vi "Traffic Control System.vi"() -> ()   [LabVIEW 2013]
panel:
  out "Red":bool
  out "Yellow":bool
  out "Green":bool
  in  "Dial 4":u16(knob) scale=0.0..9.0
  in  "Dial 3":u16(knob) scale=0.0..9.0
  in  "Dial 2":u16(knob) scale=0.0..9.0
  in  "Dial":u16(knob) scale=0.0..9.0
  in  "Yellow Timer (s)":u32
  in  "Red-Green Timer (s)":u32
  in  "Stop Button":bool
  out "Barricade Closed?":bool
  out "Barricade Open?":bool
  in  "Light State":enum16{"Red", "Green", "Yellow"}(ring)
  # "Timer Administration"
  # "Current Light State"
  # "Set the dials to correct position to enable timer modification controls"
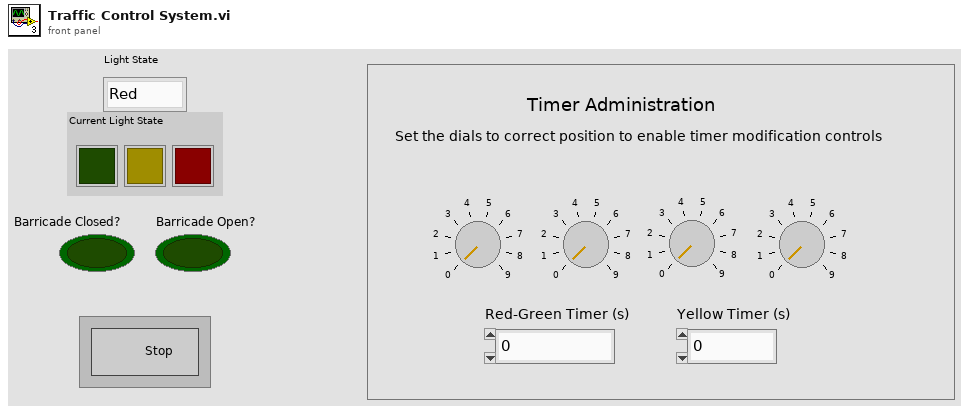
[diagram p1: front panel]
types:
  T1 = enum8{"Enabled", "Disabled", "Disabled and Grayed Out"}
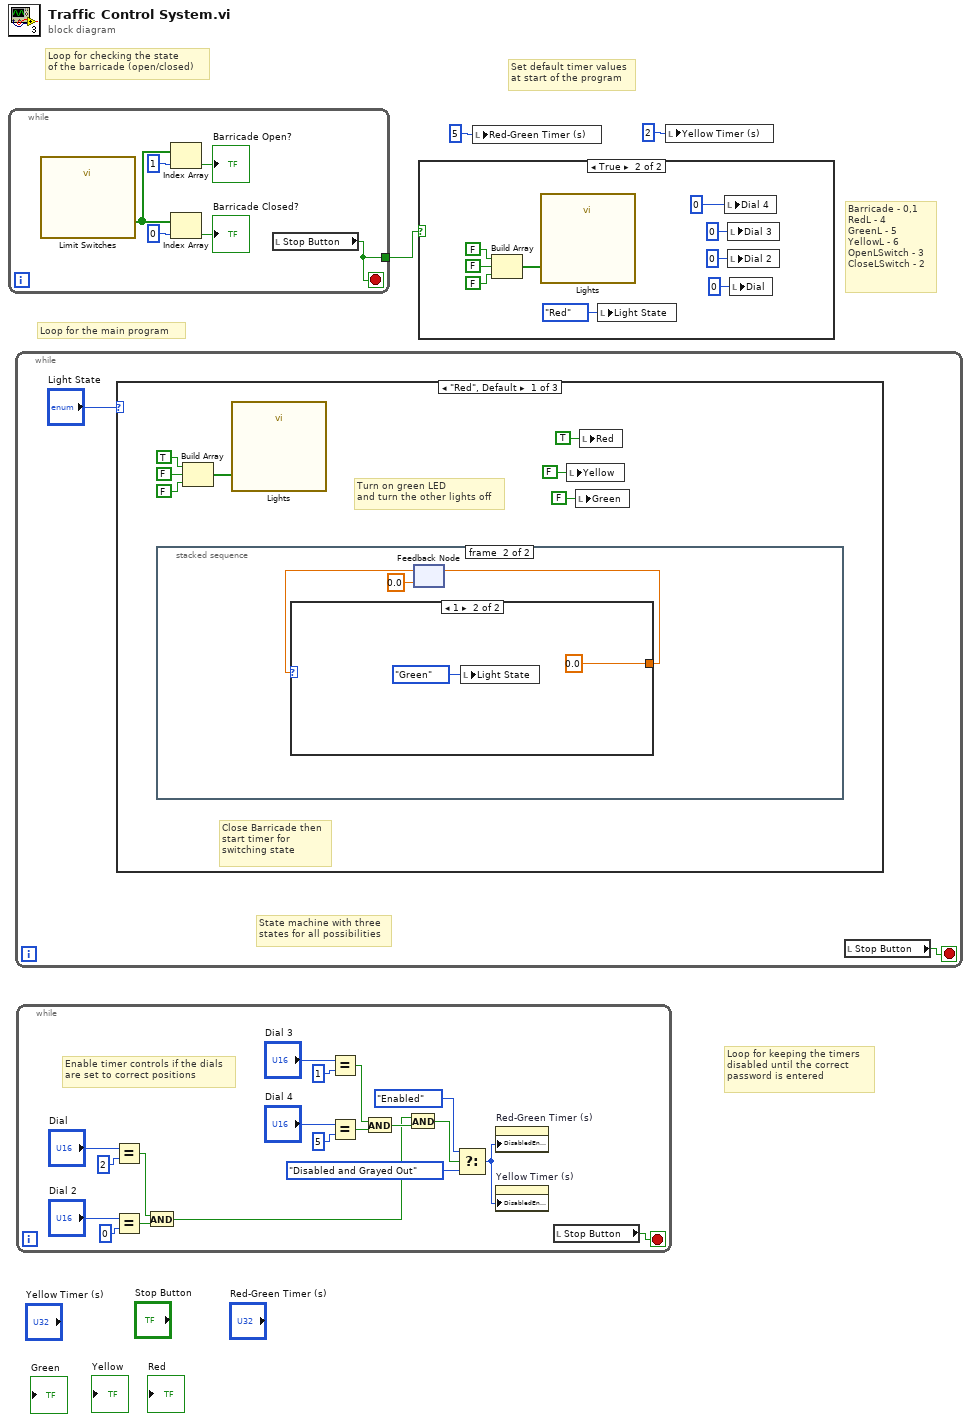
[diagram p0: block diagram]
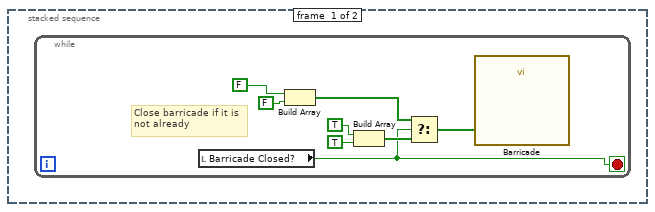
[diagram p3: hidden frame]
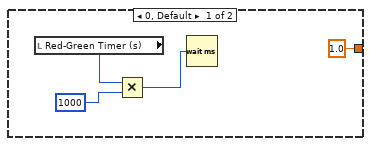
[diagram p4: hidden frame]
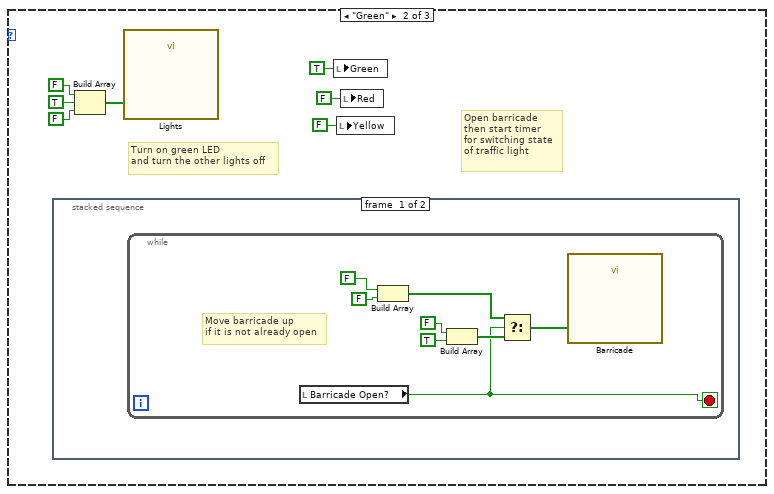
[diagram p5: hidden frame]
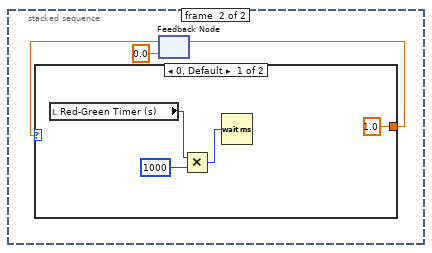
[diagram p6: hidden frame]
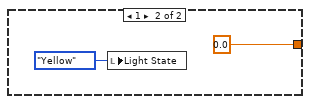
[diagram p7: hidden frame]
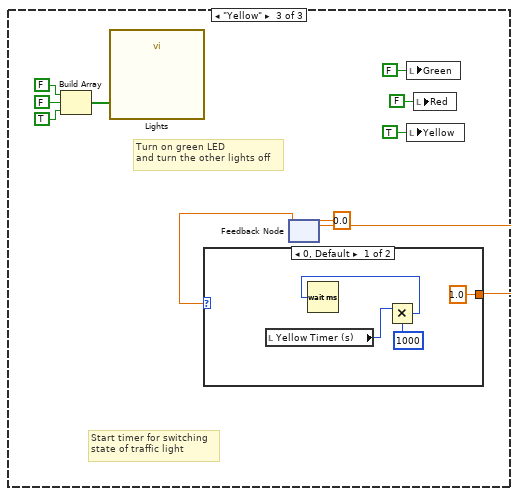
[diagram p8: hidden frame]
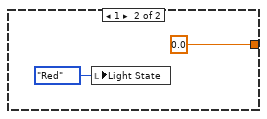
[diagram p9: hidden frame]
diagram:
  # "Loop for checking the state\nof the barricade (open/closed)"
  # "Loop for keeping the timers\ndisabled until the correct\npassword is entered"
  # "Set default timer values\nat start of the program"
  # "Loop for the main program"
  # "Barricade - 0,1\nRedL - 4\nGreenL - 5\nYellowL - 6\nOpenLSwitch - 3\nCloseLSwitch - 2"
  n1 = while {
    tunnel: [w4] -> w1
    stop <- w4 stop-if-true
    n2 = call "Limit Switches"() -> ("data"=w9:bool[])  [unwired: 17 in, 2 out]
    n3 = Index Array(array=w9, index=1) -> (element=→"Barricade Open?":bool)
    n4 = Index Array(array=w9, index=0) -> (element=→"Barricade Closed?":bool)
    n5 = local read "Stop Button"() -> (w4:bool)
  }
  n6 = while {
    stop <- w10 stop-if-true
    # "State machine with three\nstates for all possibilities"
    n7 = case shown="\"Red\", Default" "Light State" {
      frame "Red", Default {
        # "Turn on green LED\nand turn the other lights off"
        # "Close Barricade then\nstart timer for\nswitching state"
        n8 = stacked-sequence {
          frame #0 {
            n9 = while {
              stop <- w19 stop-if-true
              # "Close barricade if it is\nnot already"
              n10 = local read "Barricade Closed?"() -> (w19:bool)
              n11 = Build Array(FALSE, FALSE) -> (w21:bool[])
              n12 = Build Array(TRUE, TRUE) -> (w24:bool[])
              n13 = Select(t=w21, s=w19, f=w24) -> (s? t:f=w20:bool[])
              n14 = call "Barricade"("data"=w20) -> ()  [unwired: 17 in, 2 out]
            }
          }
          frame #1 {
            n15 = feedback #1(0.0) -> (w28:dbl)
            n16 = case shown="1" w28 {
              tunnel: [1.0 0.0] -> w29
              frame 0, Default {
                n17 = local read "Red-Green Timer (s)"() -> (w32:u32)
                n18 = Multiply(x=w32, y=u32 1000) -> (x*y=w30:u32)
                n19 = Wait (ms)(milliseconds to wait=w30) -> ()  [unwired: 1 out]
              }
              frame 1 {
                n20 = local write "Light State"(enum16{"Red", "Green", "Yellow"}."Green" ("Light State")) -> ()
              }
            }
            n21 = feedback-in #1(w29) -> ()
          }
        }
        n22 = Build Array(TRUE, FALSE, FALSE) -> (w15:bool[])
        n23 = call "Lights"("data"=w15) -> ()  [unwired: 17 in, 2 out]
        n24 = local write "Yellow"(FALSE ("Yellow")) -> ()
        n25 = local write "Green"(FALSE ("Green")) -> ()
        n26 = local write "Red"(TRUE ("Red")) -> ()
      }
      frame "Green" {
        # "Open barricade \nthen start timer\nfor switching state\nof traffic light"
        # "Turn on green LED\nand turn the other lights off"
        n27 = stacked-sequence {
          frame #0 {
            n28 = while {
              stop <- w43 stop-if-true
              # "Move barricade up\nif it is not already open"
              n29 = local read "Barricade Open?"() -> (w43:bool)
              n30 = Build Array(FALSE, FALSE) -> (w45:bool[])
              n31 = Build Array(FALSE, TRUE) -> (w48:bool[])
              n32 = Select(t=w45, s=w43, f=w48) -> (s? t:f=w44:bool[])
              n33 = call "Barricade"("data"=w44) -> ()  [unwired: 17 in, 2 out]
            }
          }
          frame #1 {
            n34 = feedback #2(0.0) -> (w53:dbl)
            n35 = case shown="0, Default" w53 {
              tunnel: [1.0 0.0] -> w51
              frame 0, Default {
                n36 = local read "Red-Green Timer (s)"() -> (w56:u32)
                n37 = Multiply(x=w56, y=u32 1000) -> (x*y=w54:u32)
                n38 = Wait (ms)(milliseconds to wait=w54) -> ()  [unwired: 1 out]
              }
              frame 1 {
                n39 = local write "Light State"(enum16{"Red", "Green", "Yellow"}."Yellow" ("Light State")) -> ()
              }
            }
            n40 = feedback-in #2(w51) -> ()
          }
        }
        n41 = Build Array(FALSE, TRUE, FALSE) -> (w39:bool[])
        n42 = call "Lights"("data"=w39) -> ()  [unwired: 17 in, 2 out]
        n43 = local write "Green"(TRUE ("Green")) -> ()
        n44 = local write "Yellow"(FALSE ("Yellow")) -> ()
        n45 = local write "Red"(FALSE ("Red")) -> ()
      }
      frame "Yellow" {
        # "Start timer for switching\nstate of traffic light"
        # "Turn on green LED\nand turn the other lights off"
        n46 = Build Array(FALSE, FALSE, TRUE) -> (w66:bool[])
        n47 = call "Lights"("data"=w66) -> ()  [unwired: 17 in, 2 out]
        n48 = feedback #3(0.0) -> (w62:dbl)
        n49 = case shown="0, Default" w62 {
          tunnel: [1.0 0.0] -> w60
          frame 0, Default {
            n50 = local read "Yellow Timer (s)"() -> (w72:u32)
            n51 = Multiply(x=w72, y=u32 1000) -> (x*y=w70:u32)
            n52 = Wait (ms)(milliseconds to wait=w70) -> ()  [unwired: 1 out]
          }
          frame 1 {
            n53 = local write "Light State"(enum16{"Red", "Green", "Yellow"}."Red" ("Light State")) -> ()
          }
        }
        n54 = feedback-in #3(w60) -> ()
        n55 = local write "Green"(FALSE ("Green")) -> ()
        n56 = local write "Yellow"(TRUE ("Yellow")) -> ()
        n57 = local write "Red"(FALSE ("Red")) -> ()
      }
    }
    n58 = local read "Stop Button"() -> (w10:bool)
  }
  n59 = while {
    stop <- w80 stop-if-true
    # "Enable timer controls if the dials\nare set to correct positions"
    n60 = Equal?(x="Dial", y=u16 2) -> (x = y?=w85:bool)
    n61 = Equal?(x="Dial 2", y=u16 0) -> (x = y?=w86:bool)
    n62 = And(x=w85, y=w86) -> (x .and. y?=w89:bool)
    n63 = Equal?(x="Dial 3", y=u16 1) -> (x = y?=w87:bool)
    n64 = Equal?(x="Dial 4", y=u16 5) -> (x = y?=w88:bool)
    n65 = And(x=w87, y=w88) -> (x .and. y?=w90:bool)
    n66 = And(x=w89, y=w90) -> (x .and. y?=w91:bool)
    n67 = Select(t=T1."Enabled" ("Disabled"), s=w91, f=T1."Disabled and Grayed Out" ("Disabled")) -> (s? t:f=w94:T1)
    n68 = property on="Red-Green Timer (s)" class="DigNum (strict)"("DisabledEnum"=w94) -> ()  [unwired: 2 in, 2 out]
    n69 = property on="Yellow Timer (s)" class="DigNum (strict)"("DisabledEnum"=w94) -> ()  [unwired: 2 in, 2 out]
    n70 = local read "Stop Button"() -> (w80:bool)
  }
  n71 = case shown="True" w1 {
    frame False {
    }
    frame True {
      n72 = Build Array(FALSE, FALSE, FALSE) -> (w101:bool[])
      n73 = call "Lights"("data"=w101) -> ()  [unwired: 17 in, 2 out]
      n74 = local write "Light State"(enum16{"Red", "Green", "Yellow"}."Red" ("Light State")) -> ()
      n75 = local write "Dial 4"(u16 0 ("Dial 4")) -> ()
      n76 = local write "Dial 3"(u16 0 ("Dial 3")) -> ()
      n77 = local write "Dial 2"(u16 0 ("Dial 2")) -> ()
      n78 = local write "Dial"(u16 0 ("Dial")) -> ()
    }
  }
  n79 = local write "Red-Green Timer (s)"(u32 5 ("Red-Green Timer")) -> ()
  n80 = local write "Yellow Timer (s)"(u32 2 ("Yellow Timer")) -> ()
